vi "MSScript_Exe_VariableDef.vi"(8 "error in (no error)":errorcluster, 9 "Expression index":i32, 11 "MSScript in":refnum<class "MSScript.lvclass">) -> (0 "Error out":errorcluster, 1 "Next expression index":i32, 3 "MSScript out":refnum<class "MSScript.lvclass">)   [LabVIEW 2018, in "MSScript.lvclass"]
uses:
  MSScript.lvclass
  MSScript.lvclass/MSScript.ctl
  MSScript_Error_(6001)VariableError.vi
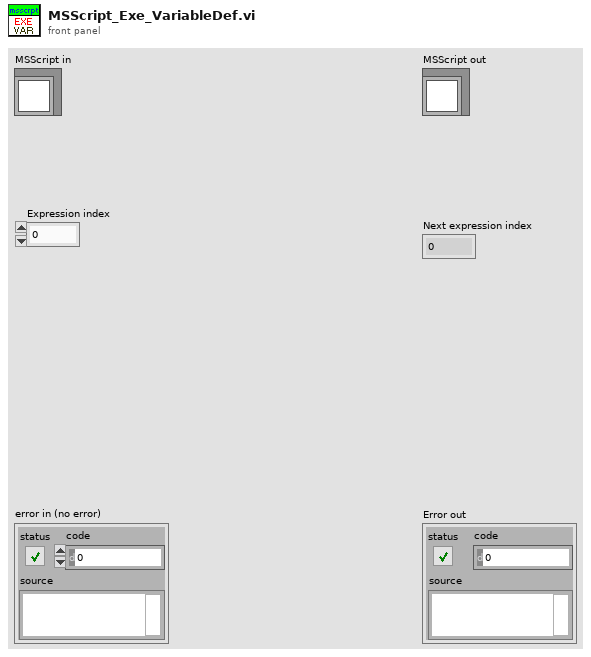
[diagram p1: front panel]
types:
  T1 = cluster{"Type":string, "NAME":cluster{"STR":string, "Start":i32}, "PARAMs":cluster{"STR":string, "Start":i32}[]}[]
  T2 = cluster{"Type":string, "NAME":cluster{"STR":string, "Start":i32}, "PARAMs":cluster{"STR":string, "Start":i32}[]}
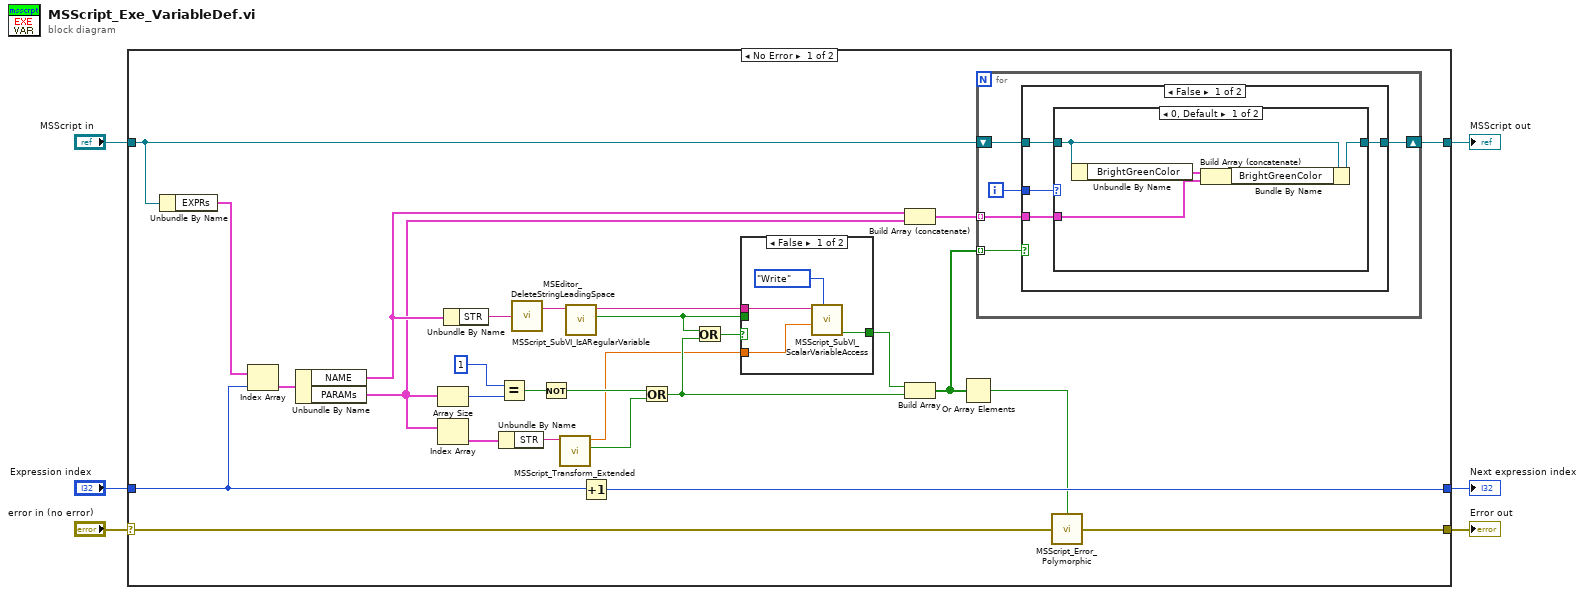
[diagram p0: block diagram]
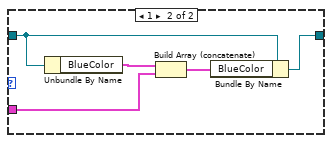
[diagram p2: hidden frame]
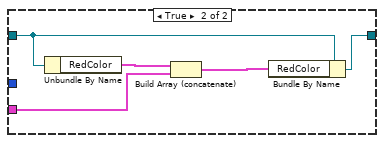
[diagram p3: hidden frame]
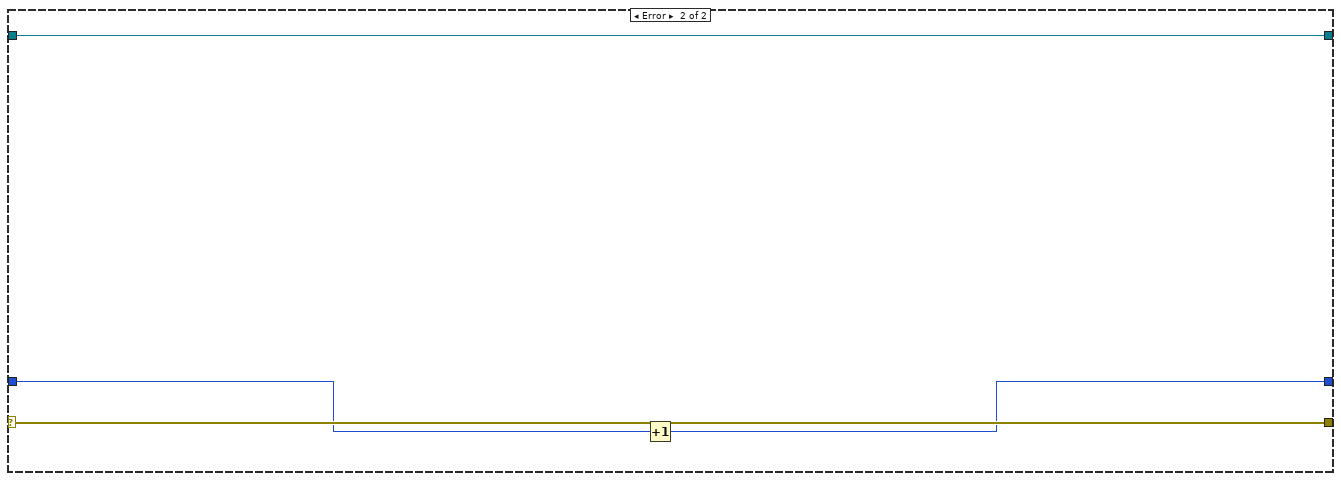
[diagram p5: hidden frame]
diagram:
  n1 = case shown="No Error" "error in (no error)" {
    selector: "error in (no error)" -> [w21 w67]
    tunnel: [w22 w65] -> w6
    tunnel: "MSScript in" -> [w12 w64]
    tunnel: "Expression index" -> [w23 w66]
    tunnel: [w20 w67] -> w2
    tunnel: [w11 w64] -> w1
    frame No Error {
      n2 = Unbundle By Name(w12) -> ("EXPRs"=w34:T1)
      n3 = Index Array(array=w34, index=w23) -> (element=w33:T2)
      n4 = Unbundle By Name(w33) -> ("NAME"=w15:cluster{"STR":string, "Start":i32}, "PARAMs"=w14:cluster{"STR":string, "Start":i32}[])
      n5 = Array Size(array=w14) -> (size(s)=w29:i32)
      n6 = Index Array(array=w14) -> (element=w24:cluster{"STR":string, "Start":i32})  [unwired: 1 in]
      n7 = Unbundle By Name(w15) -> ("STR"=w32:string)
      n8 = Equal?(x=1, y=w29) -> (x = y?=w17:bool)
      n9 = Unbundle By Name(w24) -> ("STR"=w9:string)
      n10 = call "MSEditor_DeleteStringLeadingSpace.vi"("string in"=w32) -> ("string after leading space"=w31:string)  [unwired: 1 out]
      n11 = Not(x=w17) -> (.not. x?=w16:bool)
      n12 = call "MSScript_Transform_Extended.vi"("Check_Str"=w9) -> ("Value Error?"=w7:bool, "Value Output"=w8:ext)  [unwired: 8 in, 1 out]
      n13 = call "MSScript_SubVI_IsARegularVariable.vi"("VarString in"=w31) -> ("irregular"=w19:bool, "VarString out"=w30:string)  [unwired: 6 in, 1 out]
      n14 = Increment(x=w23) -> (x+1=w22:i32)
      n15 = Or(x=w16, y=w7) -> (x .or. y?=w25:bool)
      n16 = Or(x=w19, y=w25) -> (x .or. y?=w27:bool)
      n17 = case shown="False" w27 {
        tunnel: w30 -> [w61 _]
        tunnel: [w60 w63] -> w26
        tunnel: w8 -> [w59 _]
        tunnel: w19 -> [_ w63]
        frame False {
          n18 = call "MSScript_SubVI_ScalarVariableAccess.vi"("Function (Read)"=enum16{"Init", "Write", "Read"}."Write", "VarValue"=w59, "VarName"=w61) -> ("Value Error?"=w60:bool)  [unwired: 4 in, 2 out]
        }
        frame True {
        }
      }
      n19 = Build Array (concatenate)(w15, w14) -> (w13:cluster{"STR":string, "Start":i32}[])
      n20 = Build Array(w26, w25) -> (w10:bool[])
      n21 = Or Array Elements(Boolean array=w10) -> (logical OR=w18:bool)
      n22 = for {
        tunnel: w10 -> [w37] mode=indexing
        tunnel: w13 -> [w36] mode=indexing
        shift-right: [w38] -> w11
        shift-left: w12 -> [w39]
        i -> [w35]
        n23 = case shown="False" w37 {
          tunnel: w39 -> [w41 w58]
          tunnel: [w42 w57] -> w38
          tunnel: w36 -> [w40 w55]
          tunnel: w35 -> [w43 _]
          frame False {
            n24 = case shown="0, Default" w43 {
              tunnel: [w47 w52] -> w42
              tunnel: w41 -> [w48 w53]
              tunnel: w40 -> [w45 w50]
              frame 0, Default {
                n25 = Unbundle By Name(w48) -> ("BrightGreenColor"=w46:cluster{"STR":string, "Start":i32}[])
                n26 = Build Array (concatenate)(w46, w45) -> (w44:cluster{"STR":string, "Start":i32}[])
                n27 = Bundle By Name(cluster=w48, "BrightGreenColor"=w44) -> (w47:refnum<class "MSScript.lvclass">)
              }
              frame 1 {
                n28 = Unbundle By Name(w53) -> ("BlueColor"=w51:cluster{"STR":string, "Start":i32}[])
                n29 = Build Array (concatenate)(w51, w50) -> (w49:cluster{"STR":string, "Start":i32}[])
                n30 = Bundle By Name(cluster=w53, "BlueColor"=w49) -> (w52:refnum<class "MSScript.lvclass">)
              }
            }
          }
          frame True {
            n31 = Unbundle By Name(w58) -> ("RedColor"=w56:cluster{"STR":string, "Start":i32}[])
            n32 = Build Array (concatenate)(w56, w55) -> (w54:cluster{"STR":string, "Start":i32}[])
            n33 = Bundle By Name(cluster=w58, "RedColor"=w54) -> (w57:refnum<class "MSScript.lvclass">)
          }
        }
      }
      n34 = call-poly "MSScript_Error_Polymorphic.vi"("error in (no error)"=w21, "ErrBoolean"=w18) -> ("error out"=w20:errorcluster)
    }
    frame Error {
      n35 = Increment(x=w66) -> (x+1=w65:i32)
    }
  }
  "Next expression index" <- w6
  "Error out" <- w2
  "MSScript out" <- w1
